vi "VCS Get Port Name Selection.vi"(0 "device in":T1={"deviceName"="EPOS2", "protocolStackName"="MAXON SERIAL V2", "interfaceName"="USB", "portName"=""}, 5 "startOfSelection":i32, 11 "error in (no error)":errorcluster) -> (4 "device out":T1={"deviceName"="EPOS2", "protocolStackName"="MAXON SERIAL V2", "interfaceName"="USB", "portName"=""}, 6 "endOfSelection":i32, 8 "portNameSel":string, 15 "error out":errorcluster)   [LabVIEW 2019, in "maxonEPOS.lvlib"]
doc: "<B>VCS Get Port Name Selection</B> returns all available port names."
uses:
  Examples/maxonEPOS.lvlib
  Resources/EposCmd.dll
  Resources/EposCmd64.dll
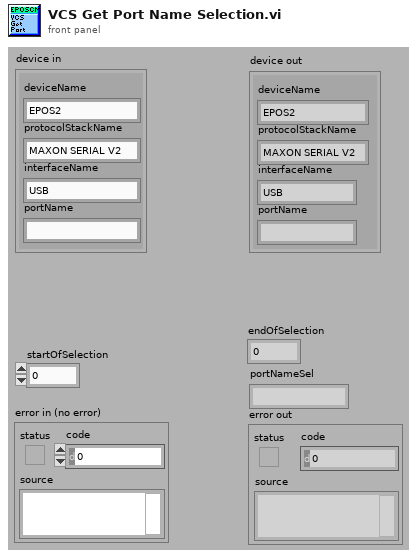
[diagram p1: front panel]
types:
  T1 = cluster{"deviceName":string, "protocolStackName":string, "interfaceName":string, "portName":string}
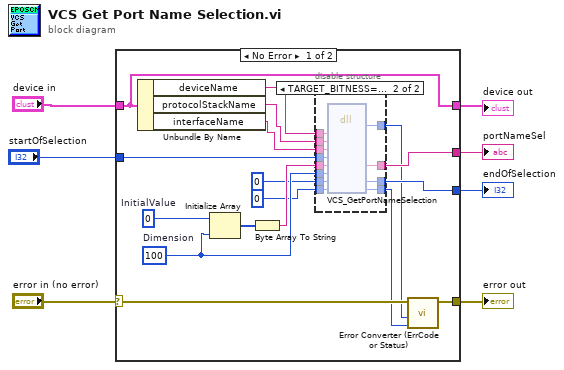
[diagram p0: block diagram]
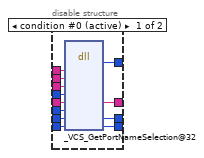
[diagram p2: hidden frame]
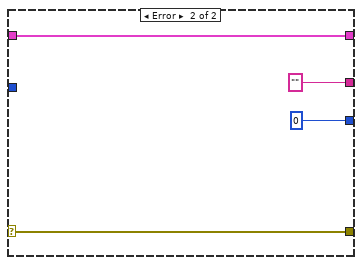
[diagram p3: hidden frame]
diagram:
  n1 = case shown="No Error" "error in (no error)" {
    selector: "error in (no error)" -> [w21 w52]
    tunnel: [w20 w52] -> w6
    tunnel: "startOfSelection" -> [w24 _]
    tunnel: [w23 "" ("pPortSel")] -> w3
    tunnel: [w22 0 ("pEndOfSelection")] -> w4
    tunnel: "device in" -> [w9 w51]
    tunnel: [w9 w51] -> w1
    frame No Error {
      w14 = u8 0  # InitialValue
      w12 = 100  # Dimension
      n2 = Unbundle By Name(w9) -> ("deviceName"=w18:string, "protocolStackName"=w17:string, "interfaceName"=w16:string)
      n3 = Initialize Array(w14, w12) -> (w15:u8[])
      n4 = Byte Array To String(unsigned byte array=w15) -> (string=w13:string)
      n5 = disable-structure shown="TARGET_BITNESS==64" {
        disable-tunnel: w24 -> [w36 w48]
        disable-tunnel: [w35 w47] -> w23
        disable-tunnel: [w34 w46] -> w22
        disable-tunnel: [w33 w45] -> w19
        disable-tunnel: w18 -> [w32 w44]
        disable-tunnel: w17 -> [w31 w43]
        disable-tunnel: w16 -> [w30 w42]
        disable-tunnel: w13 -> [w29 w41]
        disable-tunnel: w12 -> [w28 w40]
        disable-tunnel: 0 ("pEndOfSelection") -> [w27 w39]
        disable-tunnel: u32 0 ("pErrorCode") -> [w26 w38]
        disable-tunnel: [w25 w37] -> w8
        frame condition #0 (active) {
          n6 = dll-call lib="C:/workspace/project/scancon/sw/SSI_Tool/InstrumentsInterfaces/Motordriver/maxon EPOS/Resources/EposCmd.*" fn="_VCS_GetPortNameSelection@32"("DeviceName"=w32, "ProtocolStackName"=w31, "InterfaceName"=w30, "StartOfSelection"=w36, "pPortSel"=w29, "MaxStrSize"=w28, "pEndOfSelection"=w27, "pErrorCode"=w26) -> (w25:i32, "pPortSel"=w35:string, "pEndOfSelection"=w34:i32, "pErrorCode"=w33:u32)  [unwired: 8 in, 2 out]
        }
        frame condition #1 {
          n7 = dll-call lib="C:/setup/Resources/EposCmd64.*" fn="VCS_GetPortNameSelection" ("EposCmd.dll:_VCS_GetPortNameSelection@32")("DeviceName"=w44, "ProtocolStackName"=w43, "InterfaceName"=w42, "StartOfSelection"=w48, "pPortSel"=w41, "MaxStrSize"=w40, "pEndOfSelection"=w39, "pErrorCode"=w38) -> ("Rückgabetyp"=w37:i32, "pPortSel"=w47:string, "pEndOfSelection"=w46:i32, "pErrorCode"=w45:u32)  [unwired: 8 in, 2 out]
        }
      }
      n8 = call "Error Converter (ErrCode or Status).vi"("error code"=w19, "return type"=w8, "error in (no error)"=w21) -> ("error out"=w20:errorcluster)  [unwired: 7 in]
    }
    frame Error {
    }
  }
  "portNameSel" <- w3
  "endOfSelection" <- w4
  "error out" <- w6
  "device out" <- w1
